vi "Write wavelengths.vi"(8 "error in (no error)":errorcluster, 10 "wavelengths":dbl[](array[numeric]), 11 "DATA in":refnum<class "DATA.lvclass">) -> (0 "error out":errorcluster, 3 "DATA out":refnum<class "DATA.lvclass">)   [LabVIEW 2015, in "DATA.lvclass"]
uses:
  DATA.lvclass
  DATA.lvclass/DATA.ctl
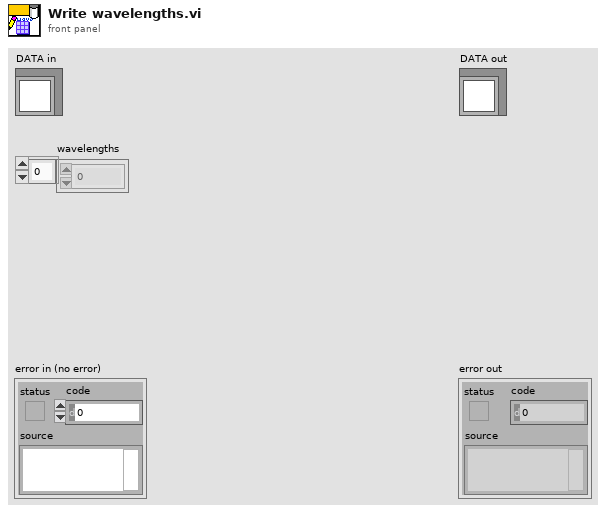
[diagram p1: front panel]
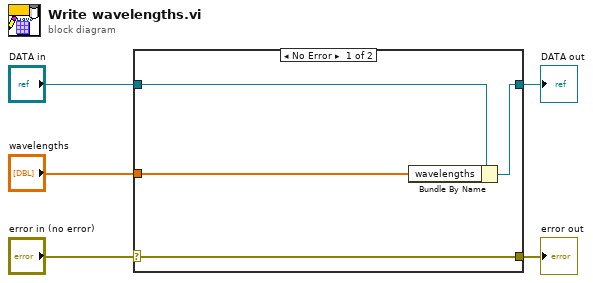
[diagram p0: block diagram]
diagram:
  n1 = case shown="No Error" "error in (no error)" {
    selector: "error in (no error)" -> [w9 w10]
    tunnel: [w9 w10] -> w4
    tunnel: [w7 w11] -> w2
    tunnel: "DATA in" -> [w8 w11]
    tunnel: "wavelengths" -> [w6 _]
    frame No Error {
      n2 = Bundle By Name(cluster=w8, "wavelengths"=w6) -> (w7:refnum<class "DATA.lvclass">)
    }
    frame Error {
    }
  }
  "error out" <- w4
  "DATA out" <- w2
